vi "Enable Heating.vi"(8 "error in (no error)":errorcluster, 10 "Ramp Rate (deg C / second)":dbl, 11 "Temperature Set Point (deg C)":dbl) -> (0 "error out":errorcluster)   [LabVIEW 2018, in "Thermal Chamber Response Simulator.lvlib"]
doc: "Enable Heating in the AE.\n____\nDelacor QMH Thermal Chamber Examples 4.0.0.21\nCopyright (c) 2018, Delacor"
uses:
  Thermal Chamber Response Simulator.lvlib
  Action--enum.ctl
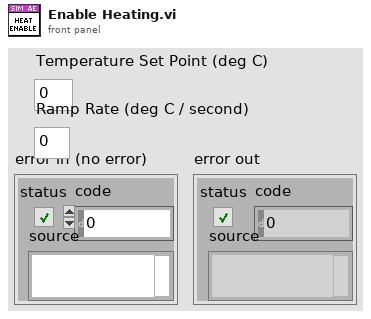
[diagram p1: front panel]
types:
  T1 = typedef "Thermal Chamber Response Simulator.lvlib/Action--enum.ctl" = enum16{"Initialize", "Set Temperature Required", "Set Ramp Rate", "Get Status", "Disable Heater", "Enable Heater", "Exit Application"}
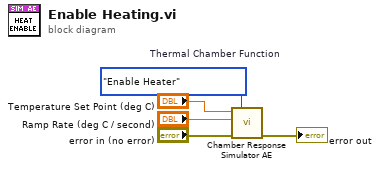
[diagram p0: block diagram]
diagram:
  w1 = Action--enum."Enable Heater"  # Thermal Chamber Function
  n1 = call "Chamber Response Simulator AE.vi"("Thermal Chamber Function"=w1, "error in (no error)"="error in (no error)", "Ramp Rate in"="Ramp Rate (deg C / second)", "Temperature Set Point in"="Temperature Set Point (deg C)") -> ("error out"=→"error out":errorcluster)  [unwired: 2 in, 5 out]
